vi "ComputeRadialProfile.vi"(6 "center":cluster{"X":sgl, "Y":sgl}, 8 "radius":sgl=32.0, 9 "radialsteps":i32=128, 10 "angularSteps":i32=64, 11 "tracker":u64) -> (2 "output":sgl[](array[numeric]), 3 "tracker":u64)   [LabVIEW 2011]
uses:
  TrackerDLL.vi
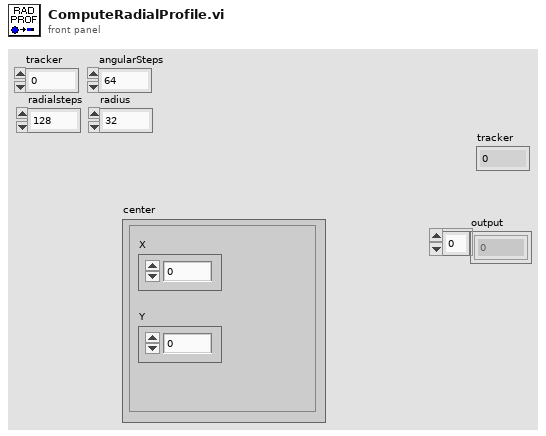
[diagram p1: front panel]
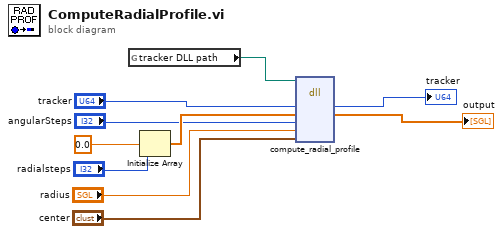
[diagram p0: block diagram]
diagram:
  n1 = global read "TrackerDLL.vi" "tracker DLL path"() -> (w10:path)
  n2 = Initialize Array(sgl 0.0 ("element"), "radialsteps") -> (w6:sgl[])
  n3 = dll-call lib="D:/jcnossen1/cudaqi-tracker/cudatrack-labview/cputrack.dll" fn="compute_radial_profile"(path in=w10, "tracker"="tracker", "output"=w6, "angularSteps"="angularSteps", "radius"="radius", "center"="center") -> ("tracker"=→"tracker":u64, "output"=→"output":sgl[])  [unwired: 6 in, 2 out]
